vi "Send Launch Server.vi"(5 "Subscriber Enqueuer":refnum<class "Message Enqueuer.lvclass">, 6 "Receive Server Enqueuer Handler":refnum<class "WebSocket Server-Service Enqueuer Msg.lvclass">, 7 "Priority":T2=enum."Normal" caption="Message Priority (Normal)", 8 "error in (no error)":errorcluster, 9 "Handshake timeout (5000 ms)":i32=5000, 10 "Listener Settings":T1={"resolve remote address (T)"=TRUE, "timeout ms (-1)"=-1, "net address"=0, "port"=6163}, 11 "Message Enqueuer in":refnum<class "Message Enqueuer.lvclass">) -> (0 "error out":errorcluster, 3 "Message Enqueuer out":refnum<class "Message Enqueuer.lvclass">)   [LabVIEW 2016, in "WebSocket Actors.lvlib" / "Launch Server Msg.lvclass"]
doc: "Sends the <b>WebSocket Actors.lvlib:Launch Server Msg.lvclass</b> message.\n\nThis message will call <b>Launch Server.vi</b> on the <b>WebSocket Actors.lvlib:WebSocket Server Manager.lvclass</b> actor.\n\n<b>Launch Server.vi Description</b>\nThis method launches a server leistening on at a specified port and interface address as detailed in the \"Listener Settings\" input. If the server is already running at that port or on the specified interface the method sends just the server enqueuer ro the client. If the server is not running it will be launched."
uses:
  Launch Server Msg.lvclass
  <vilib>/ActorFramework/Message Enqueuer/Message Enqueuer.lvclass
  <vilib>/ActorFramework/Message Enqueuer/Message Priority.ctl
  WebSocket Server/typedefs/Listener Settings.ctl
  Abstract Messages/WebSocket Server-Service Enqueuer Msg/WebSocket Server-Service Enqueuer Msg.lvclass
  C:/Program Files (x86)/National Instruments/LabVIEW 2016/vi.lib/ActorFramework/Message/Message.lvclass
  Launch Server Msg.lvclass/Launch Server Msg.ctl
  <vilib>/ActorFramework/Message Enqueuer/Message Enqueuer.lvclass/Message Enqueuer.ctl
  <vilib>/ActorFramework/Message Priority Queue/Priority Enqueue.vi
  WebSocket Server/WebSocket Server.lvclass
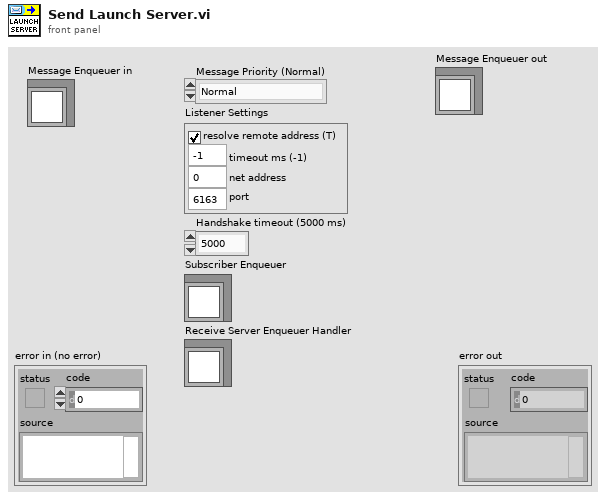
[diagram p1: front panel]
types:
  T1 = typedef "WebSocket Actors.lvlib/WebSocket Server.lvclass/Listener Settings.ctl" = cluster{"resolve remote address (T)":bool, "timeout ms (-1)":i32, "net address":u32, "port":u16}
  T2 = typedef "Actor Framework.lvlib/Message Enqueuer.lvclass/Message Priority.ctl" = enum16{"Low", "Normal", "High"}
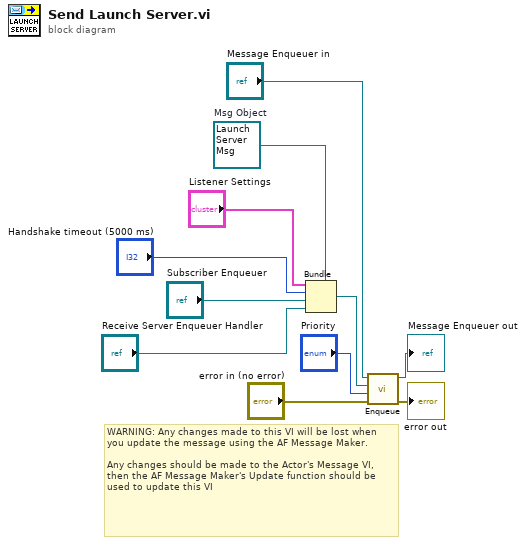
[diagram p0: block diagram]
diagram:
  w7 = refnum<class "Launch Server Msg.lvclass"> refnum  # Msg Object
  # "WARNING: Any changes made to this VI will be lost when you update the message using the AF Message Maker.\n\nAny changes should be made to the Actor's Message VI, then the AF Message Maker's Update function should be used to update this VI"
  n1 = Bundle(cluster=w7, "Listener Settings", "Handshake timeout (5000 ms)", "Subscriber Enqueuer", "Receive Server Enqueuer Handler") -> (w2:refnum<class "Launch Server Msg.lvclass">)
  n2 = call <vilib>:"Enqueue.vi"("error in (no error)"="error in (no error)", "Message Priority (Normal)"="Priority", "Message"=w2, "Message Enqueuer in"="Message Enqueuer in") -> ("error out"=→"error out":errorcluster, "Message Enqueuer out"=→"Message Enqueuer out":refnum<class "Message Enqueuer.lvclass">)  [unwired: 6 in]
